vi "delete.vi"(8 "error in (no error)":errorcluster) -> (0 "error out":errorcluster, 3 "DVR value":T1)   [LabVIEW 2018, in "main.lvlib" / "app_data.lvlib"]
uses:
  app_data.lvlib
  library_variable.vi
  app_data.ctl
  core/core_data/chessboard_index.ctl
  core/core_data/core_data.lvlib
  core/core_data/completed_tour.ctl
  core/core_data/core_data.ctl
panel:
  # "Development\ncontrols/indicators useful for development and testing, but which are not outputs of the VI"
  # "Input\nInputs to the VI"
  # "Output\nOutputs of the VI"
  # "Description\n\nBlank VI with error handling case. \n\nSummarize the use of this VI in this space."
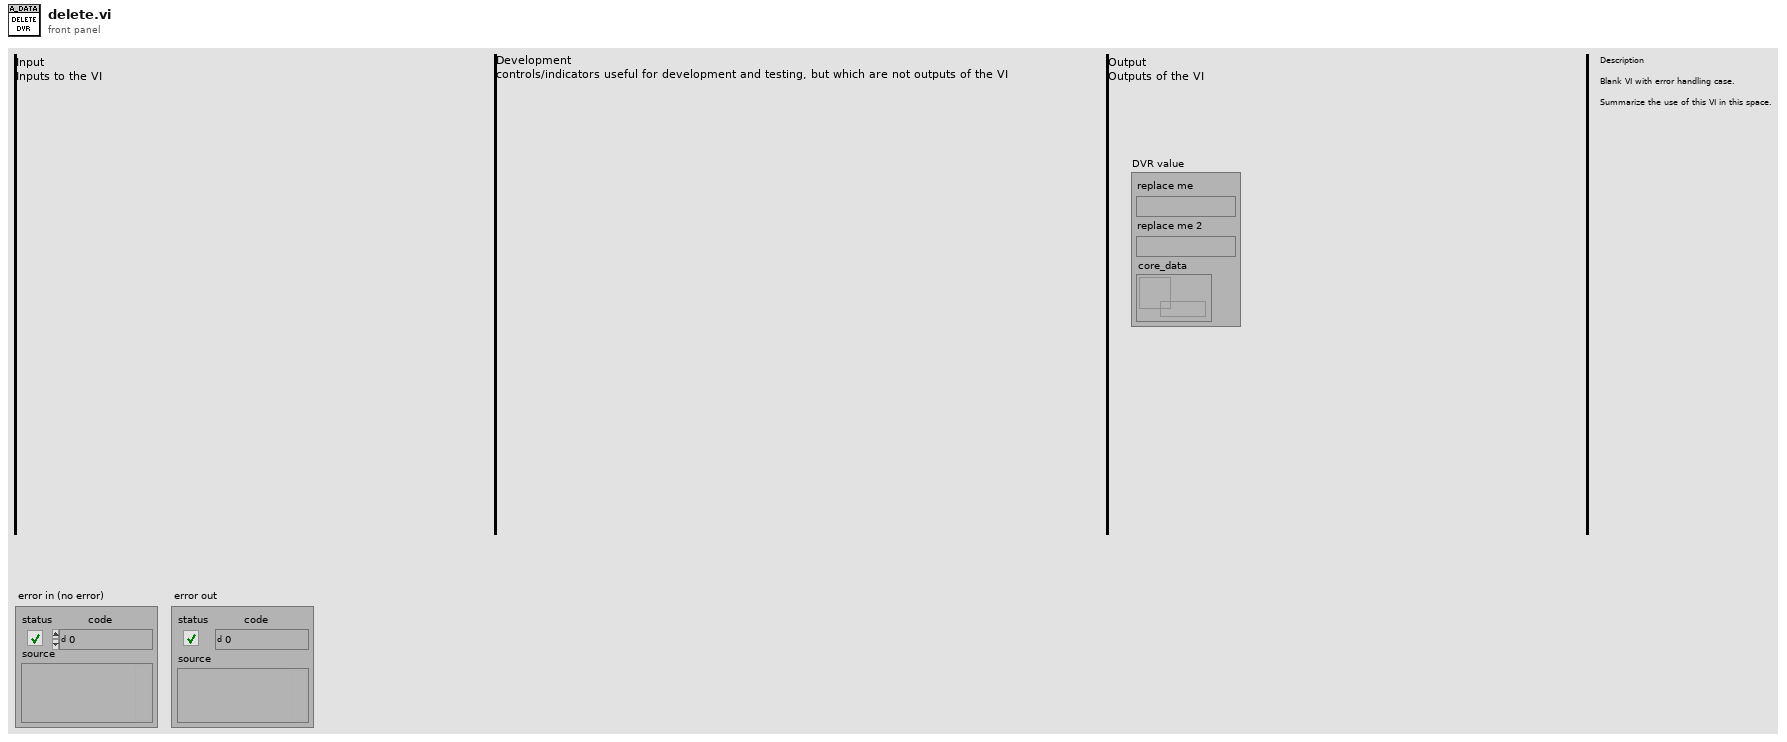
[diagram p1: front panel]
types:
  T1 = typedef "main.lvlib/app_data.lvlib/app_data.ctl" = cluster{"replace me":string, "replace me 2":string, "core_data":refnum<data-value>}
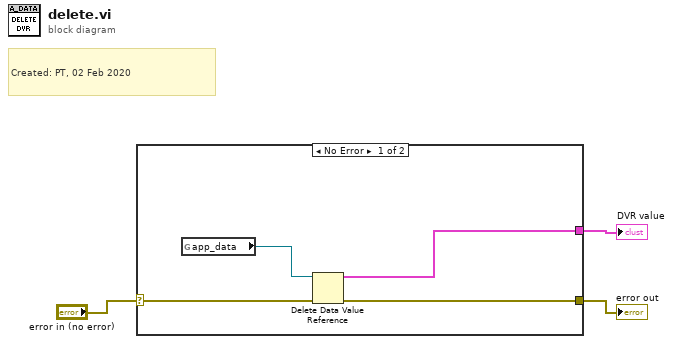
[diagram p0: block diagram]
diagram:
  # "Created: PT, 02 Feb 2020"
  n1 = case shown="No Error" "error in (no error)" {
    selector: "error in (no error)" -> [w7 w8]
    tunnel: [w6 w8] -> w2
    tunnel: [w5 _] -> w1
    frame No Error {
      n2 = global read "library_variable.vi" "app_data"() -> (w4:refnum<data-value>)
      n3 = Delete Data Value Reference(data value reference=w4, error in=w7) -> (data value=w5:T1, error out=w6:errorcluster)
    }
    frame Error {
    }
  }
  "error out" <- w2
  "DVR value" <- w1
